vi "try wavewform.vi"() -> ()   [LabVIEW 2020]
uses:
  <vilib>/measure/NI_MABase.lvlib
panel:
  in  "frequency":dbl=10.0 format="%0.2p"
  out "Waveform Chart":waveform(dbl)(graph)
  in  "stop 2":bool
  in  "stop":bool
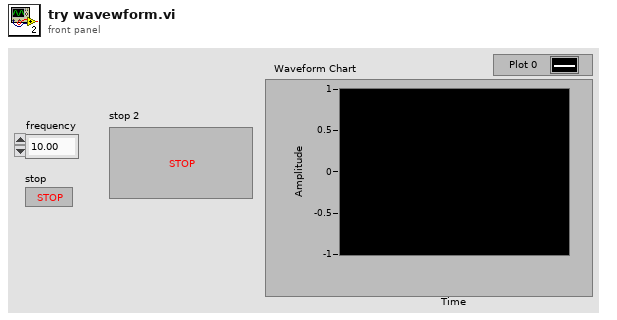
[diagram p1: front panel]
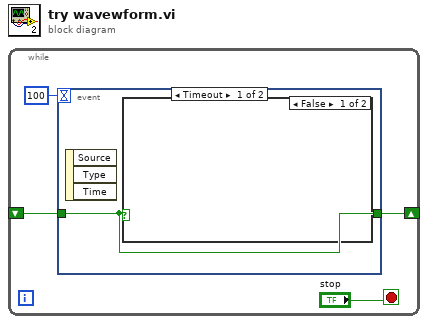
[diagram p0: block diagram]
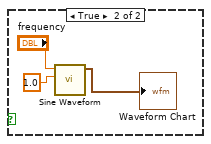
[diagram p2: hidden frame]
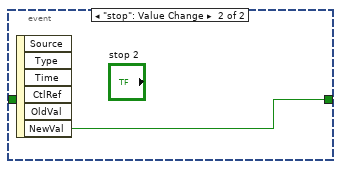
[diagram p3: hidden frame]
diagram:
  n1 = while {
    shift-right: [w1] -> _
    shift-left: _ -> [w2]
    stop <- "stop" stop-if-true
    n2 = event shown="[0] Timeout" {
      selector: _ -> [_ _]
      dyn-events: _ -> [_ _]
      timeout: 100 -> [_ _]
      tunnel: w2 -> [w5 _]
      tunnel: [w5 w9] -> w1
      event Timeout {
        n3 = event-data() -> ()  [unwired: 1 in, 3 out]
        n4 = case shown="False" w5 {
          frame False {
          }
          frame True {
            n5 = call <vilib>:"Sine Waveform.vi"("amplitude"=1.0, "frequency"="frequency") -> ("signal out"=→"Waveform Chart":waveform(dbl))  [unwired: 8 in, 1 out]
          }
        }
      }
      event "stop": Value Change {
        n6 = event-data() -> ("NewVal"=w9:bool)  [unwired: 1 in, 5 out]
      }
    }
  }
